vi "MultiTauMerge.vi"(9 "AC length":i32, 10 "Time Step":dbl, 11 "Data in":dbl[][](array[numeric])) -> (0 "Tau Times":dbl[](array[numeric]), 1 "Time Array":dbl[][](array[numeric]), 3 "XY Graph":cluster{dbl[], "Data out":dbl[]}(graph))   [LabVIEW 2022 SP3]
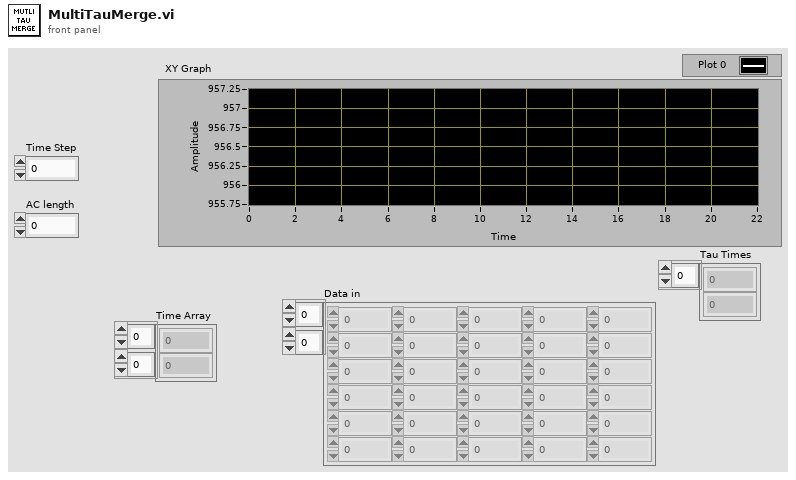
[diagram p1: front panel]
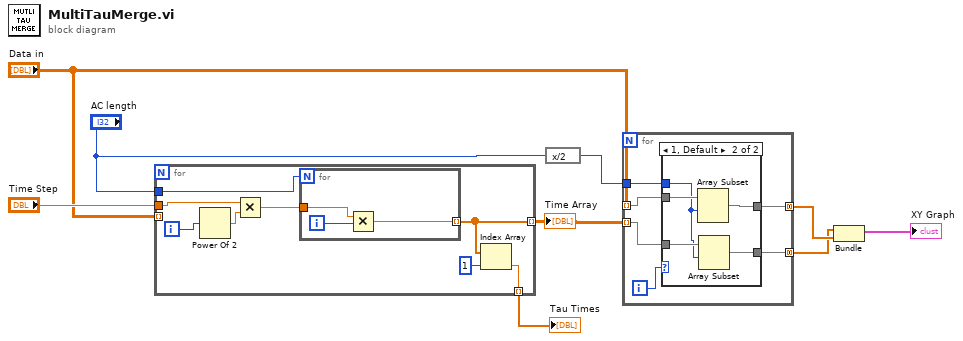
[diagram p0: block diagram]
diagram:
  n1 = for {
    tunnel: "Time Step" -> [w15]
    tunnel: "AC length" -> [w14]
    tunnel: [w11] -> w5 mode=indexing
    tunnel: "Data in" -> [_] mode=indexing
    tunnel: [w10] -> w1 mode=indexing
    i -> [w17]
    n2 = Power Of 2(x=w17) -> (2^x=w16:dbl)
    n3 = Multiply(x=w15, y=w16) -> (x*y=w13:dbl)
    n4 = for {
      N: w14 -> [_]
      tunnel: w13 -> [w19]
      tunnel: [w18] -> w11 mode=indexing
      i -> [w20]
      n5 = Multiply(x=w19, y=w20) -> (x*y=w18:dbl)
    }
    n6 = Index Array(array=w11, index=1) -> (element=w10:dbl)
  }
  "Time Array" <- w5
  "Tau Times" <- w1
  n7 = expression code="x/2"("AC length") -> (w7:i32)
  n8 = for {
    tunnel: [w25] -> w4 mode=concatenating
    tunnel: "Data in" -> [w24] mode=indexing
    tunnel: w5 -> [w23] mode=indexing
    tunnel: [w22] -> w8 mode=concatenating
    tunnel: w7 -> [w21]
    i -> [w26]
    n9 = case shown="1, Default" w26 {
      tunnel: [w27 w30] -> w25
      tunnel: w24 -> [w28 w33]
      tunnel: w23 -> [w27 w32]
      tunnel: [w28 w31] -> w22
      tunnel: w21 -> [_ w29]
      frame 0 {
      }
      frame 1, Default {
        n10 = Array Subset(array=w33, index=w29) -> (w31:dbl[])  [unwired: 1 in]
        n11 = Array Subset(array=w32, index=w29) -> (w30:dbl[])  [unwired: 1 in]
      }
    }
  }
  n12 = Bundle(w4, "Data in"=w8) -> (→"XY Graph":cluster{dbl[], "Data in":dbl[]})  [unwired: 1 in]
